vi "Send.vi"(7 "Format (Text)":T1, 8 "error in (no error)":errorcluster, 9 "Timeout ms (1000)":i32=1000, 10 "Payload":string, 11 "WebSocket Client in":refnum<class "WebSocket Client.lvclass">) -> (0 "error out":errorcluster, 3 "WebSocket Client out":refnum<class "WebSocket Client.lvclass">)   [LabVIEW 2020, in "HTTP Server.lvlib" / "WebSocket Client.lvclass"]
uses:
  WebSocket Client.lvclass
  WebSocket Client.lvclass/WebSocket Client.ctl
  Lock Type.ctl
  WebSocket Format.ctl
  HTTP Server.lvlib
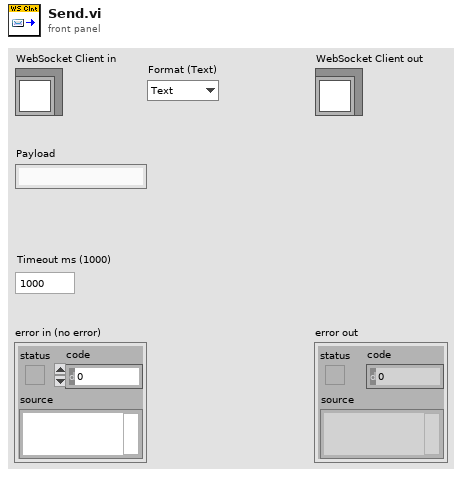
[diagram p1: front panel]
types:
  T1 = typedef "HTTP Server.lvlib/WebSocket Format.ctl" = enum16{"Text", "Binary"}
  T2 = typedef "HTTP Server.lvlib/WebSocket Client.lvclass/Lock Type.ctl" = enum16{"Read", "Write"}
  T3 = typedef "HTTP Server.lvlib/WebSocket Client.lvclass/OpCode.ctl" = enum8{"Continuation", "Text", "Binary", "Reserved3", "Reserved4", "Reserved5", "Reserved6", "Reserved7", "Close", "Ping", "Pong", "ReservedB", "ReservedC", "ReservedD", "ReservedE", "ReservedF"}
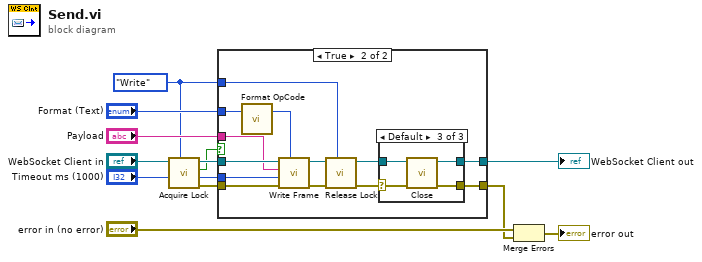
[diagram p0: block diagram]
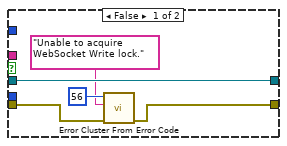
[diagram p2: hidden frame]
diagram:
  w4 = Lock_Type."Write" ("Lock Type")
  n1 = call "Acquire Lock.vi"("Lock Type"=w4, "Timeout ms"="Timeout ms (1000)", "WebSocket Client in"="WebSocket Client in") -> ("error out"=w13:errorcluster, "Remaining  Timeout"=w7:i32, "Acquired"=w6:bool, "WebSocket Client out"=w10:refnum<class "WebSocket Client.lvclass">)  [unwired: 5 in]
  n2 = case shown="True" w6 {
    tunnel: w13 -> [w18 w31]
    tunnel: w10 -> [w15 w29]
    tunnel: [w15 w19] -> w9
    tunnel: "Payload" -> [_ w28]
    tunnel: w7 -> [_ w27]
    tunnel: "Format (Text)" -> [_ w26]
    tunnel: w4 -> [_ w22]
    tunnel: [w16 w21] -> w1
    frame False {
      n3 = call <vilib>:"Error Cluster From Error Code.vi"("error in (no error)"=w18, "error message (\"\")"="Unable to acquire WebSocket Write lock.", "error code (0)"=56) -> ("error out"=w16:errorcluster)  [unwired: 6 in]
    }
    frame True {
      n4 = call "Format OpCode.vi"("Format"=w26) -> ("OpCode"=w25:T3)  [unwired: 6 in]
      n5 = call "Write Frame.vi"("OpCode"=w25, "error in (no error)"=w31, "Timeout ms"=w27, "Payload"=w28, "WebSocket Client in"=w29) -> ("error out"=w30:errorcluster, "WebSocket Client out"=w23:refnum<class "WebSocket Client.lvclass">)  [unwired: 4 in, 1 out]
      n6 = call "Release Lock.vi"("Lock Type"=w22, "error in (no error)"=w30, "WebSocket Client in"=w23) -> ("error out"=w24:errorcluster, "WebSocket Client out"=w20:refnum<class "WebSocket Client.lvclass">)  [unwired: 7 in]
      n7 = case shown="Default" w24 {
        selector: w24 -> [w32 _ w38]
        tunnel: [w32 _ w37] -> w21
        tunnel: w20 -> [w33 w34 w36]
        tunnel: [w33 w34 w35] -> w19
        frame No Error {
        }
        frame Error {
        }
        frame Default {
          n8 = call "Close.vi"("error in (no error)"=w38, "WebSocket Client in"=w36) -> ("error out"=w37:errorcluster, "WebSocket Client out"=w35:refnum<class "WebSocket Client.lvclass">)  [unwired: 8 in]
        }
      }
    }
  }
  "WebSocket Client out" <- w9
  n9 = Merge Errors("error in (no error)", w1) -> (→"error out":errorcluster)
